vi "abort ps control.vi"   [LabVIEW 2019]
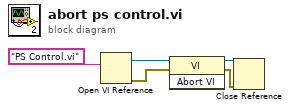
[diagram p0: block diagram]
diagram:
  n1 = Open VI Reference(vi path="PS Control.vi") -> (vi reference=w4:refnum<vi>, error out=w5:errorcluster)  [unwired: 5 in]
  n2 = invoke class="VI" method="Abort VI"(reference=w4, error in=w5) -> (reference out=w2:refnum<vi>, error out=w3:errorcluster)  [unwired: 1 in, 1 out]
  n3 = Close Reference(reference=w2, error in (no error)=w3) -> ()  [unwired: 1 out]
